vi "Start Server.vi"(8 "error in (no error)":errorcluster, 11 "gRPC Server in":refnum<class "Streamer_server.lvclass">) -> (0 "error out":errorcluster, 2 "Listening Port":i32, 3 "gRPC Server out":refnum<class "Streamer_server.lvclass">)   [LabVIEW 2019, in "Streamer_server.lvlib" / "Streamer_server.lvclass"]
uses:
  Streamer_server.lvclass
  Streamer_server.lvclass/Streamer_server.ctl
  <vilib>/gRPC/LabVIEW gRPC Library/gprc-lvsupport-release.lvlib
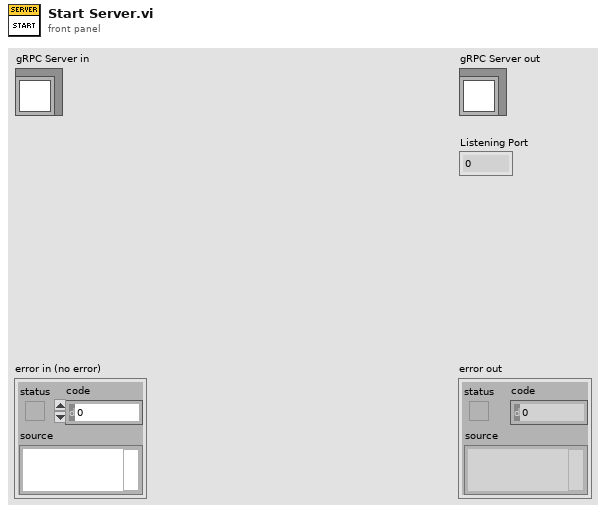
[diagram p1: front panel]
types:
  T1 = typedef "gprc-lvsupport-release.lvlib/grpcId.ctl" = u64
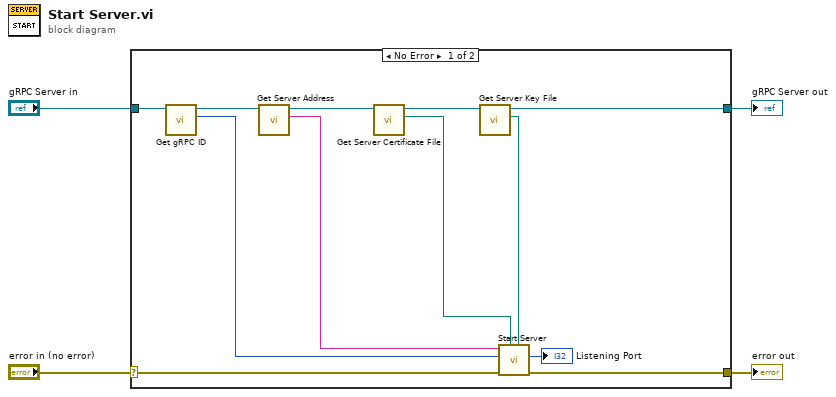
[diagram p0: block diagram]
diagram:
  n1 = case shown="No Error" "error in (no error)" {
    selector: "error in (no error)" -> [w16 w18]
    tunnel: [w6 w18] -> w3
    tunnel: [w7 w17] -> w1
    tunnel: "gRPC Server in" -> [w14 w17]
    frame No Error {
      n2 = call "Get gRPC ID.vi"("OOP Server in"=w14) -> ("gRPC ID"=w12:T1, "OOP Server out"=w13:refnum<class "Streamer_server.lvclass">)  [unwired: 9 in]
      n3 = call "Get Server Address.vi"("OOP Server in"=w13) -> ("Server Address"=w15:string, "OOP Server out"=w11:refnum<class "Streamer_server.lvclass">)  [unwired: 9 in]
      n4 = call "Get Server Certificate File.vi"("OOP Server in"=w11) -> ("Server Certificate File (.crt)"=w10:path, "OOP Server out"=w9:refnum<class "Streamer_server.lvclass">)  [unwired: 9 in]
      n5 = call "Get Server Key File.vi"("OOP Server in"=w9) -> ("Server Key File (.key)"=w8:path, "OOP Server out"=w7:refnum<class "Streamer_server.lvclass">)  [unwired: 9 in]
      n6 = call <vilib>:"Start Server.vi"("Server Key File (.key)"=w8, "Server Certificate File (.crt)"=w10, "error in (no error)"=w16, "Server Id"=w12, "Server Address"=w15) -> ("error out"=w6:errorcluster, "Listening Port"=→"Listening Port":i32)  [unwired: 4 in, 1 out]
    }
    frame Error {
    }
  }
  "error out" <- w3
  "gRPC Server out" <- w1
